vi "Annotation_Save.vi"(5 "Class Names":string[](array[string]), 7 "Annotations (CWH)":T1[](array[typedef]) {"BBox"."x" format="%#_4p"; "BBox"."y" format="%#_4p"; "BBox"."w" format="%#_4p"; "BBox"."h" format="%#_4p"}, 8 "error in (no error)":errorcluster, 11 "appended path":path) -> (0 "error out":errorcluster)   [LabVIEW 2020]
uses:
  <vilib>/Ngene/Deep Learning Toolkit/Toolkit/NN_Data/API/Data/Detection_Types/NN_BBox_Annotation.ctl
  <vilib>/Ngene/Deep Learning Toolkit/Toolkit/NN_Data/API/Data/Detection_Types/NN_BBox.ctl
  <vilib>/Utility/error.llb/whitespace.ctl
  <vilib>/Ngene/Deep Learning Toolkit/Toolkit/NN_Data/API/Data/Detection_Types/NN_BBox_Format_Conversion_Direction.ctl
  <vilib>/Ngene/Deep Learning Toolkit/Toolkit/Deep_Learning_Toolkit_by_Ngene.lvlib
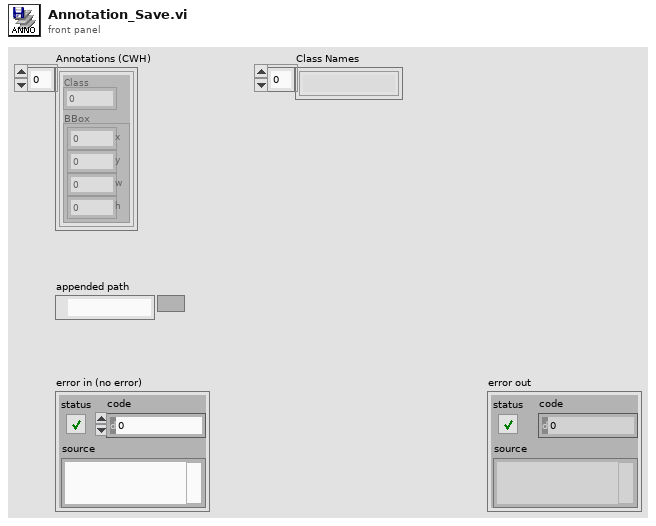
[diagram p1: front panel]
types:
  T1 = typedef "Deep_Learning_Toolkit_by_Ngene.lvlib/NN_BBox_Annotation.ctl" = cluster{"Class":i32, "BBox":T2}
  T2 = typedef "Deep_Learning_Toolkit_by_Ngene.lvlib/NN_BBox.ctl" = cluster{"x":sgl, "y":sgl, "w":sgl, "h":sgl}
  T3 = typedef "Deep_Learning_Toolkit_by_Ngene.lvlib/NN_BBox_Format_Conversion_Direction.ctl" = enum16{"SS_to_CWH", "CWH_to_SS"}
  T4 = typedef "whitespace.ctl" = u16
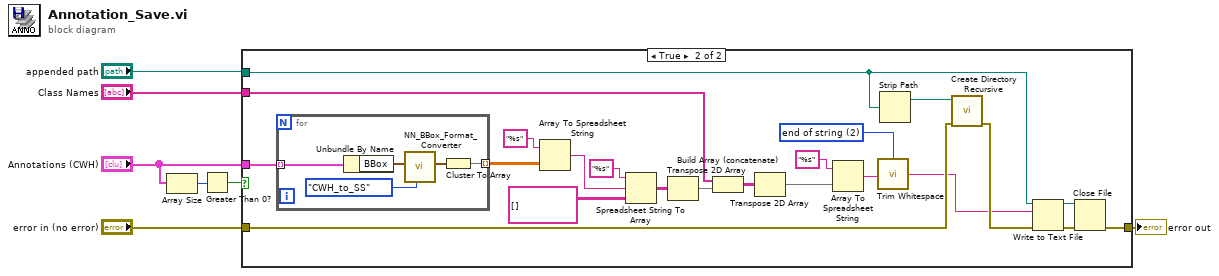
[diagram p0: block diagram]
diagram:
  n1 = Array Size(array="Annotations (CWH)") -> (size(s)=w2:i32)
  n2 = Greater Than 0?(x=w2) -> (x > 0?=w1:bool)
  n3 = case shown="True" w1 {
    tunnel: [w8 w30] -> w7
    tunnel: "error in (no error)" -> [w8 w13]
    tunnel: "appended path" -> [_ w14]
    tunnel: "Annotations (CWH)" -> [_ w18]
    tunnel: "Class Names" -> [_ w16]
    frame False {
    }
    frame True {
      w10 = T4 2 items=["both", "start of string", "end of string"] ("location (both)")
      n4 = for {
        tunnel: w18 -> [w35] mode=indexing
        tunnel: [w31] -> w17 mode=indexing
        n5 = Unbundle By Name(w35) -> ("BBox"=w34:T2)
        n6 = call <vilib>:"NN_BBox_Format_Converter.vi"("Conversion_Direction"=NN_BBox_Format_Conversion_Direction."CWH_to_SS" ("Format_Transform"), "BBox in"=w34) -> ("BBox out"=w32:T2)  [unwired: 9 in]
        n7 = Cluster To Array(cluster=w32) -> (array=w31:sgl[])
      }
      n8 = Array To Spreadsheet String(array=w17, 3:"%s" ("format string")) -> (spreadsheet string=w21:string)  [unwired: 1 in]
      n9 = Spreadsheet String To Array(format string="%s" ("format (%.3f)"), spreadsheet string=w21, array type (2D Dbl)=string[][] []) -> (array=w23:string[][])  [unwired: 1 in]
      n10 = Transpose 2D Array(2D array=w23) -> (transposed array=w24:string[][])
      n11 = Build Array (concatenate)(w16, w24) -> (w25:string[][])
      n12 = Transpose 2D Array(2D array=w25) -> (transposed array=w27:string[][])
      n13 = Array To Spreadsheet String(array=w27, 3:"%s" ("format string")) -> (spreadsheet string=w11:string)  [unwired: 1 in]
      n14 = call <vilib>:"Trim Whitespace.vi"("string"=w11, "location (both)"=w10) -> ("trimmed string"=w9:string)
      n15 = Strip Path(path=w14) -> (stripped path=w15:path)  [unwired: 1 out]
      n16 = call <vilib>:"Create Directory Recursive.vi"("error in (no error)"=w13, "directory"=w15) -> ("error out"=w12:errorcluster)  [unwired: 3 in, 2 out]
      n17 = Write to Text File(file (use dialog)=w14, text=w9, error in=w12) -> (refnum out=w28:refnum<file>, error out=w29:errorcluster)  [unwired: 1 in, 1 out]
      n18 = Close File(refnum=w28, error in=w29) -> (error out=w30:errorcluster)  [unwired: 1 out]
    }
  }
  "error out" <- w7
